vi "ProcessWithoutOutput.vi"() -> ()   [LabVIEW 2013]
uses:
  <vilib>/Instr/_visa.llb/VISA Configure Serial Port (Instr).vi
panel:
  out "Standardabweichung":dbl
  out "Ready":bool
  out "Line Received":bool
  in  "Serial Input":refnum<visa-resource-name>="COM5"
  in  "Smoothing":bool
  out "Einfallswinkel":dbl(knob) scale=-90.0..90.0
  in  "Gaussian Fit":bool
  in  "Stop Button":bool
  # "Osten"
  # "Westen"
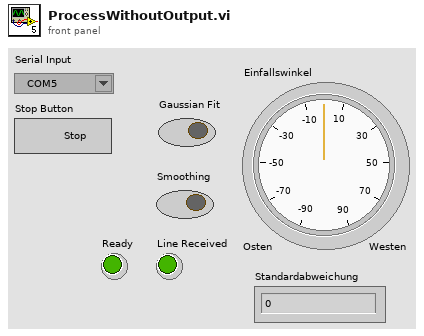
[diagram p1: front panel]
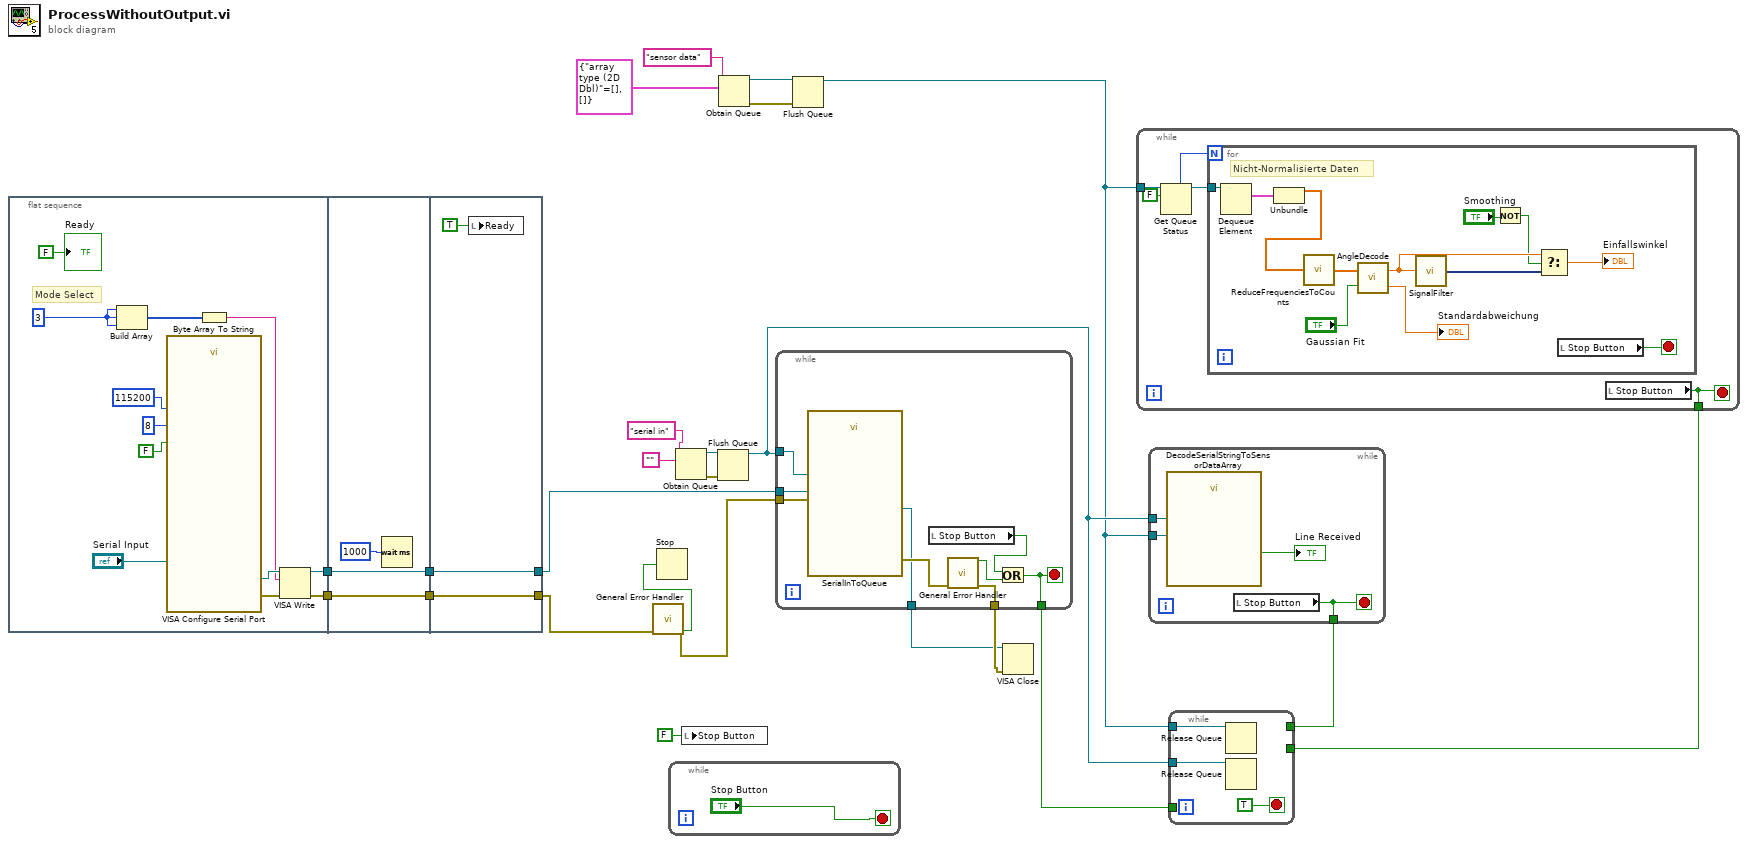
[diagram p0: block diagram]
diagram:
  n1 = flat-sequence {
    tunnel: [w29] -> w2
    tunnel: [w28] -> w1
    tunnel: [w38] -> w4
    tunnel: [w37] -> w3
    tunnel: w2 -> [w38]
    tunnel: w1 -> [w37]
    tunnel: [w40] -> w5
    tunnel: [w41] -> w6
    tunnel: w4 -> [w41]
    tunnel: w3 -> [w40]
    frame #0 {
      w31 = u8 3 ("number")
      # "Mode Select"
      n2 = Build Array(w31, w31, w31) -> (w32:u8[])
      n3 = call-poly "VISA Configure Serial Port"("VISA resource name"="Serial Input", "Enable Termination\nChar (T)"=FALSE ("Enable Termination\nChar (T)"), "baud rate (9600)"=u32 115200, "data bits (8)"=u16 8) -> ("VISA resource name out"=w27:refnum<visa-resource-name>, "error out"=w26:errorcluster)  [unwired: 10 in]
      n4 = Byte Array To String(unsigned byte array=w32) -> (string=w25:string)
      n5 = VISA Write(VISA resource name=w27, write buffer=w25, error in (no error)=w26) -> (VISA resource name out=w29:refnum<visa-resource-name>, error out=w28:errorcluster)  [unwired: 1 out]
      "Ready" <- FALSE ("Ready")
    }
    frame #1 {
      n6 = Wait (ms)(milliseconds to wait=u32 1000) -> ()  [unwired: 1 out]
    }
    frame #2 {
      n7 = local write "Ready"(TRUE ("Ready")) -> ()
    }
  }
  n8 = call <vilib>:"General Error Handler.vi"("error in (no error)"=w5) -> ("error?"=w15:bool, "error out"=w16:errorcluster)  [unwired: 10 in, 3 out]
  n9 = Stop(stop? (T)=w15) -> ()
  n10 = while {
    stop <- "Stop Button" stop-if-true
  }
  n11 = Obtain Queue(name (unnamed)="serial in", element data type="") -> (queue out=w18:refnum<queue>, error out=w17:errorcluster)  [unwired: 3 in, 1 out]
  n12 = local write "Stop Button"(FALSE ("Stop Button")) -> ()
  n13 = Flush Queue(queue=w18, error in (no error)=w17) -> (queue out=w12:refnum<queue>)  [unwired: 2 out]
  n14 = Obtain Queue(name (unnamed)="sensor data", element data type=cluster{"array type (2D Dbl)":dbl[], dbl[]} {"array type (2D Dbl)"=[], []} ("output cluster")) -> (queue out=w20:refnum<queue>, error out=w19:errorcluster)  [unwired: 3 in, 1 out]
  n15 = while {
    tunnel: w6 -> [w52]
    tunnel: w12 -> [w46]
    tunnel: w16 -> [w51]
    tunnel: [w50] -> w14
    tunnel: [w45] -> w10
    tunnel: [w44] -> w7
    stop <- w45 stop-if-true
    n16 = call "SerialInToQueue.vi"("error in (no error)"=w51, "VISA resource name in"=w52, "Queue in"=w46) -> ("error out"=w49:errorcluster, "VISA resource name"=w44:refnum<visa-resource-name>)  [unwired: 5 in, 2 out]
    n17 = local read "Stop Button"() -> (w47:bool)
    n18 = call <vilib>:"General Error Handler.vi"("error in (no error)"=w49) -> ("error?"=w48:bool, "error out"=w50:errorcluster)  [unwired: 10 in, 3 out]
    n19 = Or(x=w47, y=w48) -> (x .or. y?=w45:bool)
  }
  n20 = Flush Queue(queue=w20, error in (no error)=w19) -> (queue out=w11:refnum<queue>)  [unwired: 2 out]
  n21 = VISA Close(VISA resource name=w7, error in (no error)=w14) -> ()  [unwired: 1 out]
  n22 = while {
    tunnel: w11 -> [w56]
    tunnel: [w55] -> w8
    stop <- w55 stop-if-true
    n23 = Get Queue Status(queue=w56, return elements? (F)=FALSE) -> (queue out=w53:refnum<queue>, # elements in queue=w57:i32)  [unwired: 1 in, 6 out]
    n24 = for {
      N: w57 -> [_]
      tunnel: w53 -> [w60]
      stop <- w61 stop-if-true
      # "Nicht-Normalisierte Daten"
      n25 = Dequeue Element(queue=w60) -> (element=w59:cluster{"array type (2D Dbl)":dbl[], dbl[]})  [unwired: 2 in, 3 out]
      n26 = Unbundle(w59) -> ("array type (2D Dbl)"=w62:dbl[])  [unwired: 1 out]
      n27 = call "ReduceFrequenciesToCounts.vi"("Sensor Frequencies (kHz)"=w62) -> ("Sensor Counts"=w63:dbl[])
      n28 = call "AngleDecode.vi"("Interpolate"="Gaussian Fit", "Data"=w63) -> ("Standard Deviation"=→"Standardabweichung":dbl, "Peak Angle"=w68:dbl)
      n29 = call "SignalFilter.vi"("Signal In"=w68) -> ("Filtered Signal"=w65:dynamicdata)
      n30 = Not(x="Smoothing") -> (.not. x?=w67:bool)
      n31 = Select(t=w68, s=w67, f=w65) -> (s? t:f=→"Einfallswinkel":dbl)
      n32 = local read "Stop Button"() -> (w61:bool)
    }
    n33 = local read "Stop Button"() -> (w55:bool)
  }
  n34 = while {
    tunnel: w11 -> [w73]
    tunnel: w12 -> [w71]
    tunnel: [w70] -> w9
    stop <- w70 stop-if-true
    n35 = call "DecodeSerialStringToSensorDataArray.vi"("Serial String Queue in"=w71, "Sensor Data Queue in"=w73) -> ("Line Received"=→"Line Received":bool)  [unwired: 1 out]
    n36 = local read "Stop Button"() -> (w70:bool)
  }
  n37 = while {
    tunnel: w12 -> [w75]
    tunnel: w11 -> [w74]
    tunnel: w10 -> [_]
    tunnel: w9 -> [_]
    tunnel: w8 -> [_]
    stop <- TRUE stop-if-true
    n38 = Release Queue(queue=w74) -> ()  [unwired: 2 in, 3 out]
    n39 = Release Queue(queue=w75) -> ()  [unwired: 2 in, 3 out]
  }
